vi "Analyzer2.vi"() -> ()   [LabVIEW 2014]
uses:
  <vilib>/express/express analysis/Spectral/Block/exnSpectralBlock spectral measurements RMS poly.vi
  <vilib>/express/express analysis/Spectral/Block/exnSpectralBlock spectral measurements RMS WFM.vi
  <vilib>/express/express analysis/Spectral/XNode/ExpressSpectralMeasurementsBlockNode.xnode
  <vilib>/measure/NI_MABase.lvlib
panel:
  out "magnitude":dbl[](array[numeric])
  out "Waveform Chart":waveform(dbl)(graph)
  in  "stop":bool
  out "Fourier Spect":cluster{"f0":dbl, "df":dbl, "magnitude":dbl[]}(graph)
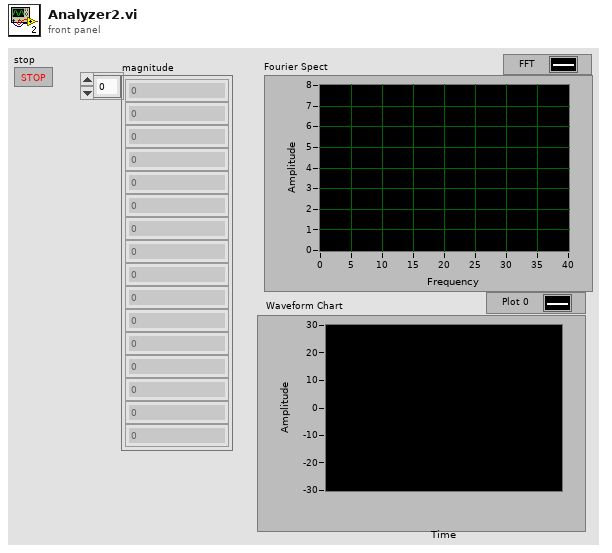
[diagram p1: front panel]
types:
  T1 = cluster{"averaging mode":u16, "weighting mode":u16, "number of averages":u32}
  T2 = cluster{"dB On (F)":bool, "unwrap phase (F)":bool, "convert to degree (F)":bool}
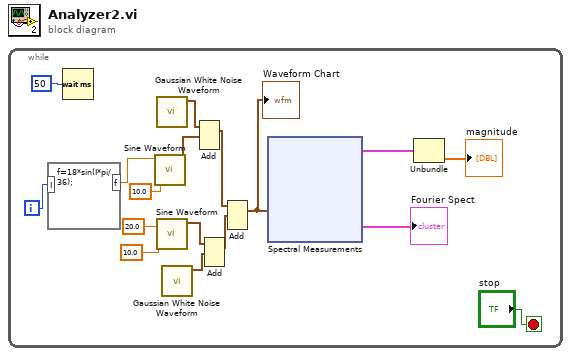
[diagram p0: block diagram]
diagram:
  n1 = while {
    i -> [w14]
    stop <- "stop" stop-if-true
    n2 = formula code="f=18*sin(I*pi/36);"("I"=w14) -> ("f"=w15:dbl)
    n3 = Wait (ms)(milliseconds to wait=u32 50) -> ()  [unwired: 1 out]
    n4 = call <vilib>:"Sine Waveform.vi"("amplitude"=10.0, "frequency"=w15) -> ("signal out"=w6:waveform(dbl))  [unwired: 8 in, 1 out]
    n5 = call <vilib>:"Gaussian White Noise Waveform.vi"() -> ("signal out"=w7:waveform(dbl))  [unwired: 10 in, 1 out]
    n6 = call <vilib>:"Sine Waveform.vi"("amplitude"=10.0, "frequency"=20.0) -> ("signal out"=w2:waveform(dbl))  [unwired: 8 in, 1 out]
    n7 = call <vilib>:"Gaussian White Noise Waveform.vi"() -> ("signal out"=w3:waveform(dbl))  [unwired: 10 in, 1 out]
    n8 = Add(1:w6, 2:w7) -> (0:w5:waveform(dbl))  [unwired: 1 in, 1 out]
    n9 = Add(1:w3, 2:w2) -> (0:w1:waveform(dbl))  [unwired: 1 in, 1 out]
    n10 = Add(1:w1, 2:w5) -> (0:w4:waveform(dbl))  [unwired: 1 in, 1 out]
    "Waveform Chart" <- w4
    n11 = xnode "Spectral Measurements"("Signals"=w4) -> ("FFT - (RMS)"=w9:cluster{"f0":dbl, "df":dbl, "magnitude":dbl[]})  [unwired: 1 in, 2 out]
    "Fourier Spect" <- w9
    n12 = Unbundle(w9) -> ("magnitude"=→"magnitude":dbl[])  [unwired: 2 out]
  }
